vi "LastStepMsgParser.vi"(6 "Arr Refnum":refnum<vi>, 7 "Out MSG Names":string[](array[string]), 8 "old msg counter":i32, 9 "Codes":i32[](array[numeric]), 10 "Msg Array":T1(array[cluster])) -> (2 "code":i32[](array[numeric]), 3 "current msg counter":i32)   [LabVIEW 2019]
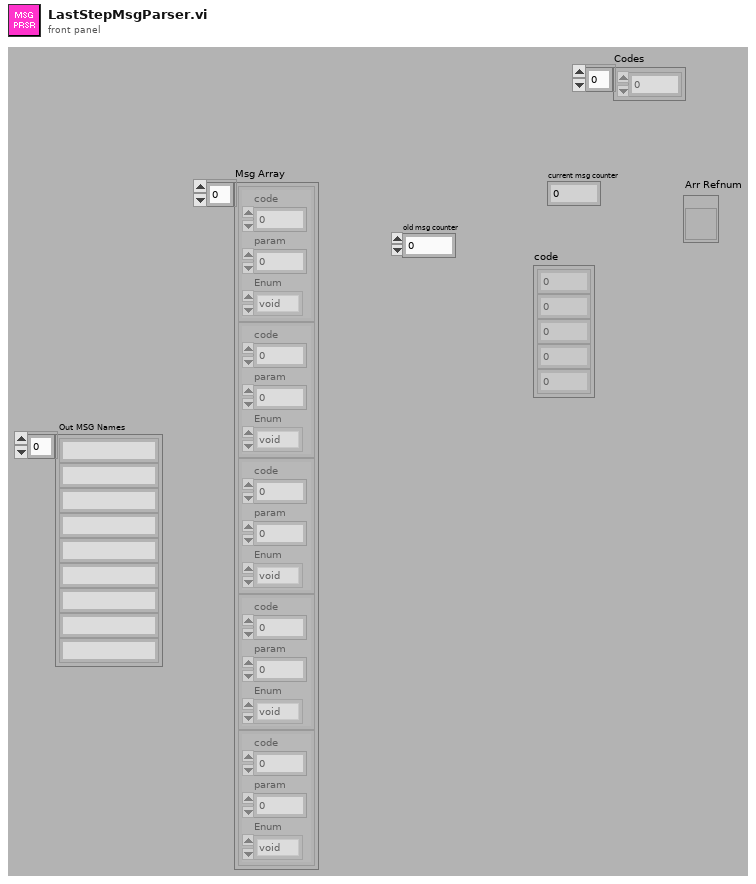
[diagram p1: front panel]
types:
  T1 = cluster{"code":i16, "param":i32, "Enum":enum16{"void", "byte", "int", "float"}}[]
  T2 = cluster{"code":i32, "param":i32, "Enum":enum16{"void", "byte", "int", "float"}}
  T3 = cluster{"Сообщение":string, "Значение":string, "Тип":enum16{"void", "byte", "int", "float"}}[]
  T4 = cluster{"Сообщение":string, "Значение":string, "Тип":enum16{"void", "byte", "int", "float"}}
  T5 = cluster{"code":i16, "param":i32, "Enum":enum16{"void", "byte", "int", "float"}}
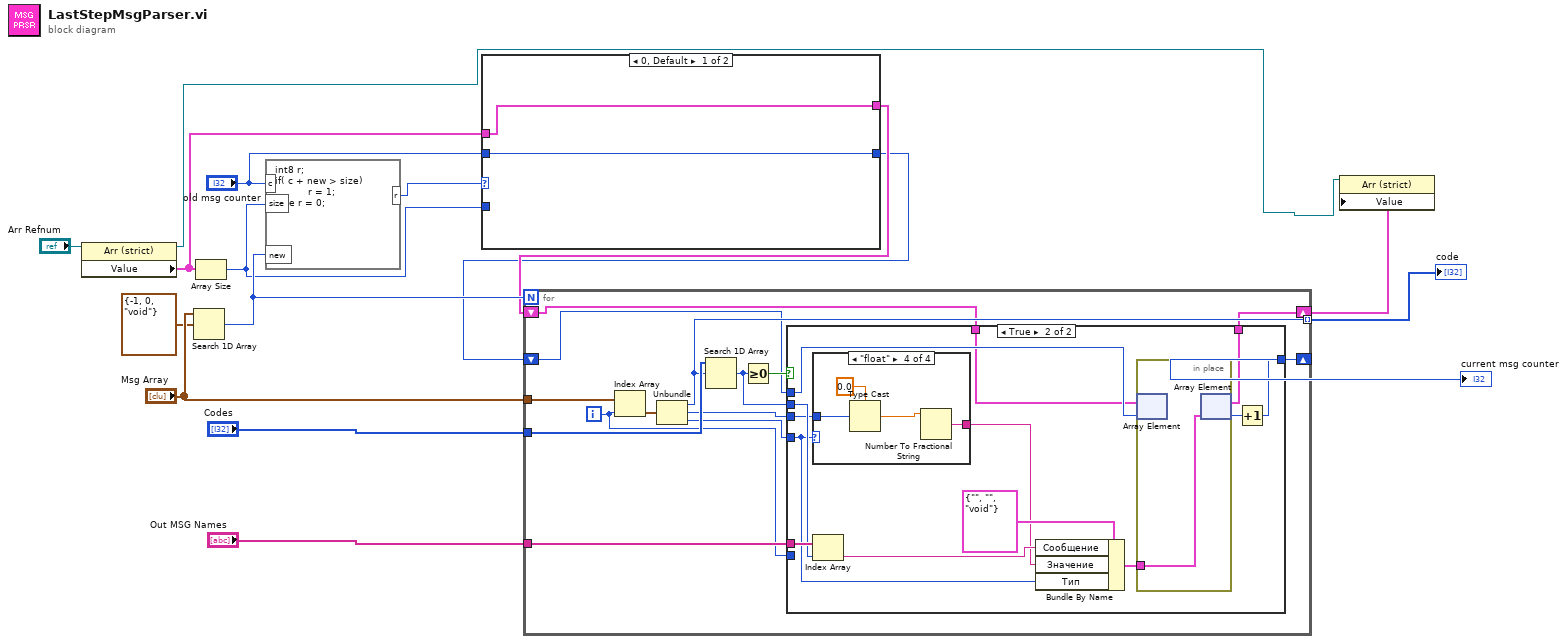
[diagram p0: block diagram]
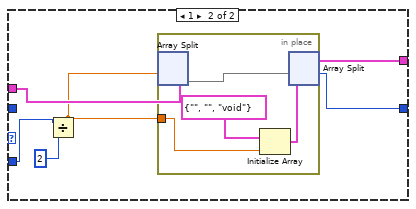
[diagram p2: hidden frame]
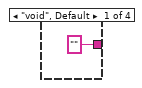
[diagram p4: hidden frame]
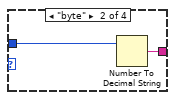
[diagram p5: hidden frame]
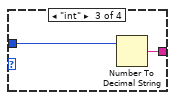
[diagram p6: hidden frame]
diagram:
  n1 = property class="Arr (strict)"(reference="Arr Refnum") -> (reference out=w5:refnum<vi>, "Value"=w8:T3)  [unwired: 1 in, 1 out]
  n2 = Search 1D Array(1D array="Msg Array", element=T2 {"code"=-1, "param"=0, "Enum"=enum."void"} ("Cluster")) -> (index of element=w7:i32)  [unwired: 1 in]
  n3 = Array Size(array=w8) -> (size(s)=w4:i32)
  n4 = formula code="int8 r;\nif( c + new > size)\n           r = 1;\nelse r = 0;"("c"="old msg counter", "size"=w4, "new"=w7) -> ("r"=w9:i8)
  n5 = case shown="0, Default" w9 {
    tunnel: w8 -> [w18 w22]
    tunnel: w4 -> [_ w24]
    tunnel: [w18 w20] -> w6
    tunnel: "old msg counter" -> [w17 _]
    tunnel: [w17 w19] -> w2
    frame 0, Default {
    }
    frame 1 {
      n6 = Divide(x=w24, y=2) -> (x/y=w21:dbl)
      n7 = in-place {
        in-place-border: w21 -> [w27]
        n8 = in-place-split #1(w22, w21) -> (w28:T3)  [unwired: 1 out]
        n9 = Initialize Array(T4 {"Сообщение"="", "Значение"="", "Тип"=enum."void"} ("Cluster"), w27) -> (w25:T3)
        n10 = in-place-split #1(w28, w25) -> (w20:T3, w19:i32)
      }
    }
  }
  n11 = for {
    N: w7 -> [_]
    tunnel: "Msg Array" -> [w37]
    tunnel: [w33] -> w15 mode=indexing
    tunnel: "Codes" -> [w40]
    tunnel: "Out MSG Names" -> [w39]
    shift-right: [w31] -> w11
    shift-left: w2 -> [w32]
    shift-right: [w29] -> w1
    shift-left: w6 -> [w30]
    i -> [w36]
    n12 = Index Array(array=w37, index=w36) -> (element=w35:T5)
    n13 = Unbundle(w35) -> ("code"=w33:i16, "param"=w38:i32, "Enum"=w34:enum16{"void", "byte", "int", "float"})
    n14 = Search 1D Array(1D array=w40, element=w33) -> (index of element=w41:i32)  [unwired: 1 in]
    n15 = Greater Or Equal To 0?(x=w41) -> (x >= 0?=w42:bool)
    n16 = case shown="True" w42 {
      tunnel: w39 -> [_ w57]
      tunnel: w41 -> [_ w56]
      tunnel: w38 -> [_ w55]
      tunnel: w36 -> [_ _]
      tunnel: w34 -> [_ w51]
      tunnel: w32 -> [w44 w48]
      tunnel: [w44 w49] -> w31
      tunnel: w30 -> [w43 w47]
      tunnel: [w43 w46] -> w29
      frame False {
      }
      frame True {
        n17 = case shown="\"float\"" w51 {
          tunnel: w55 -> [_ w61 w63 w67]
          tunnel: ["" ("decimal integer string") w60 w62 w64] -> w52
          frame "void", Default {
          }
          frame "byte" {
            n18 = Number To Decimal String(number=w61) -> (decimal integer string=w60:string)  [unwired: 1 in]
          }
          frame "int" {
            n19 = Number To Decimal String(number=w63) -> (decimal integer string=w62:string)  [unwired: 1 in]
          }
          frame "float" {
            n20 = Type Cast(type=sgl 0.0 ("default (0 dbl)"), x=w67) -> (*(type *) &x=w65:sgl)
            n21 = Number To Fractional String(number=w65) -> (F-format string=w64:string)  [unwired: 3 in]
          }
        }
        n22 = Index Array(array=w57, index=w56) -> (element=w53:string)
        n23 = Bundle By Name(cluster=T4 {"Сообщение"="", "Значение"="", "Тип"=enum."void"} ("Cluster"), "Сообщение"=w53, "Значение"=w52, "Тип"=w51) -> (w50:T4)
        n24 = in-place {
          in-place-border: w50 -> [w58]
          n25 = in-place-array #2(w47, w48) -> ()  [unwired: 1 out]
          n26 = in-place-array #2(w58) -> (w46:T3, w45:i32)
        }
        n27 = Increment(x=w45) -> (x+1=w49:i32)
      }
    }
  }
  "code" <- w15
  "current msg counter" <- w11
  n28 = property class="Arr (strict)"(reference=w5, "Value"=w1) -> ()  [unwired: 1 in, 2 out]
